vi "dfd_NStage MRate Set Filtering Mode.vi"(6 "filtering mode":T6=2 items=["No Rate Change", "Interpolation", "Decimation"], 8 "error in (no error)":errorcluster, 11 "multirate filter in":T1[](array[typedef]) {"mMRate_SumWl" min=1 max=32 step=1; "mMRate_InputIwl" min=1 max=32 step=1; "mMRate_GainWl" min=1 max=32 step=1; "mMRate_OutputWl" min=1 max=32 step=1; "mMRate_InputWl" min=1 max=32 step=1; "mMRate_CoefWl" min=1 max=32 step=1; "mMRate_Mode" items=["Default"=-1, "No Rate Change"=0, "Interpolation"=1, "Decimation"=2, "Interpolated"=3, "Rational"=4]}) -> (0 "error out":errorcluster, 3 "multirate filter out":T1[](array[typedef]) {"mMRate_SumWl" min=1 max=32 step=1; "mMRate_InputIwl" min=1 max=32 step=1; "mMRate_GainWl" min=1 max=32 step=1; "mMRate_OutputWl" min=1 max=32 step=1; "mMRate_InputWl" min=1 max=32 step=1; "mMRate_CoefWl" min=1 max=32 step=1; "mMRate_Mode" items=["Default"=-1, "No Rate Change"=0, "Interpolation"=1, "Decimation"=2, "Interpolated"=3, "Rational"=4]})   [LabVIEW 2017, in "NI_DigFilterLicensed.lvlib"]
uses:
  <vilib>/addons/Digital Filter Design/NI_DigFilterLicensed.lvlib
  <vilib>/addons/Digital Filter Design/_Objects.llb/DFD Multirate Filtering Mode.ctl
  <vilib>/addons/Digital Filter Design/_Objects.llb/DFD Multirate Filter Obj.ctl
  <vilib>/addons/Digital Filter Design/_Objects.llb/DFD Multirate Mode.ctl
  <vilib>/addons/Digital Filter Design/_Objects.llb/DFD Coef Norm Type.ctl
  <vilib>/addons/Digital Filter Design/_Objects.llb/DFD Round-off Mode.ctl
  <vilib>/addons/Digital Filter Design/_Objects.llb/DFD FXP MRate Multiply Mode.ctl
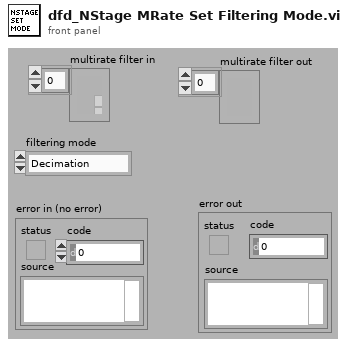
[diagram p1: front panel]
types:
  T1 = typedef "NI_DigFilterLicensed.lvlib/DFD Multirate Filter Obj.ctl" = cluster{"mMRate_Structure":enum16{"CIC", "FIR", "IIR", "Lattice"}, "mMRate_Mode":T2, "mMRate_Factor":i32, "mMRate_FIRParams":cluster{"mMRate_FIR_H":dbl[], "mMRate_FIR_IsNyquist?":bool, "mMRate_FIR_IsSymmetric?":bool}, "mMRate_CICParams":cluster{"mMRate_CIC_#Stage":i32, "mMRate_CIC_Lag":i32, "mMRate_CIC_Type":enum16{"Lowpass", "Highpass"}}, "mMRate_Order":i32, "mMRate_Version":string, "mMRate_Comments":string, "mMRate_RationalFactor":cluster{"mMRate_L":i32, "mMRate_M":i32}, "mMRate_Fs":dbl, "mMRate_Quantized?":bool, "mMRate_QFilterGain":dbl, "mMRate_CoefWl":i16, "mMRate_Scaling":cluster{"mMRate_ScaleByPowerOf2?":bool, "mMRate_ScaleType":T3}, "mMRate_InputWl":i16, "mMRate_OutputWl":i16, "mMRate_OutputMode":T4, "mMRate_MultMode":T5, "mMRate_BitPruning":bool, "mMRate_GainWl":i16, "mMRate_OutputFwl":i16, "mMRate_SumIwl":i16, "mMRate_InputIwl ":i16, "mMRate_SumWl":i16, "mMRate_CoefIwl":i16}
  T2 = typedef "NI_DigFilterLicensed.lvlib/DFD Multirate Mode.ctl" = i16
  T3 = typedef "NI_DigFilterLicensed.lvlib/DFD Coef Norm Type.ctl" = enum16{"No Norm", "Time Domain 1-Norm", "Time Domain 2-Norm", "Time Domain Inf-Norm"}
  T4 = typedef "NI_DigFilterLicensed.lvlib/DFD Round-off Mode.ctl" = enum16{"Nearest", "Truncation"}
  T5 = typedef "NI_DigFilterLicensed.lvlib/DFD FXP MRate Multiply Mode.ctl" = enum16{"Truncated", "Full"}
  T6 = typedef "NI_DigFilterLicensed.lvlib/DFD Multirate Filtering Mode.ctl" = u16
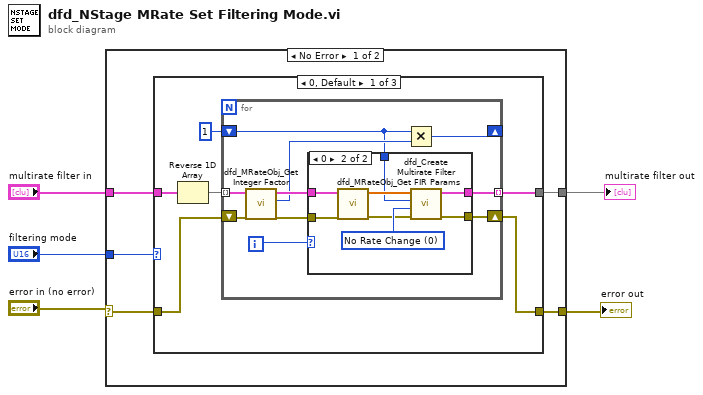
[diagram p0: block diagram]
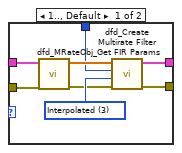
[diagram p2: hidden frame]
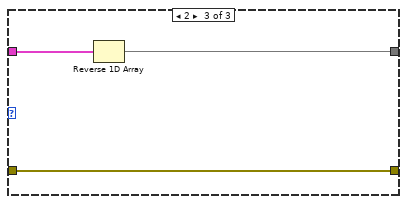
[diagram p4: hidden frame]
diagram:
  n1 = case shown="No Error" "error in (no error)" {
    selector: "error in (no error)" -> [w7 w45]
    tunnel: "filtering mode" -> [w10 _]
    tunnel: [w9 _] -> w4
    tunnel: "multirate filter in" -> [w8 _]
    tunnel: [w6 w45] -> w1
    frame No Error {
      n2 = case shown="0, Default" w10 {
        tunnel: w8 -> [w16 w41 w44]
        tunnel: [w12 w41 w43] -> w9
        tunnel: w7 -> [w14 w40 w42]
        tunnel: [w11 w40 w42] -> w6
        frame 0, Default {
          n3 = Reverse 1D Array(array=w16) -> (reversed array=w15:T1[])
          n4 = for {
            tunnel: w15 -> [w21] mode=indexing
            shift-right: [w18] -> _
            shift-left: 1 -> [w17]
            shift-right: [w23] -> w11
            shift-left: w14 -> [w24]
            tunnel: [w22] -> w12 mode=indexing
            i -> [w25]
            n5 = call <vilib>:"dfd_MRateObj_Get Integer Factor.vi"("multirate filter in"=w21) -> ("factor"=w19:i32, "dup multirate filter"=w20:T1)  [unwired: 9 out]
            n6 = case shown="0" w25 {
              tunnel: w20 -> [w32 w39]
              tunnel: w17 -> [w27 w34]
              tunnel: w24 -> [w26 w33]
              tunnel: [w30 w37] -> w23
              tunnel: [w29 w36] -> w22
              frame 1.., Default {
                w28 = T2 3 items=["Default"=-1, "No Rate Change"=0, "Interpolation"=1, "Decimation"=2, "Interpolated"=3] ("mode")
                n7 = call <vilib>:"dfd_MRateObj_Get FIR Params.vi"("multirate filter in"=w32) -> ("h(n)"=w31:dbl[])  [unwired: 1 in, 9 out]
                n8 = call <vilib>:"dfd_Create Multirate Filter.vi"("error in (no error)"=w26, "mode"=w28, "factor"=w27, "h (n)"=w31) -> ("error out"=w30:errorcluster, "multirate filter out"=w29:T1)  [unwired: 1 in, 5 out]
              }
              frame 0 {
                w35 = T2 0 items=["Default"=-1, "No Rate Change"=0, "Interpolation"=1, "Decimation"=2, "Interpolated"=3] ("mode")
                n9 = call <vilib>:"dfd_MRateObj_Get FIR Params.vi"("multirate filter in"=w39) -> ("h(n)"=w38:dbl[])  [unwired: 1 in, 9 out]
                n10 = call <vilib>:"dfd_Create Multirate Filter.vi"("error in (no error)"=w33, "mode"=w35, "factor"=w34, "h (n)"=w38) -> ("error out"=w37:errorcluster, "multirate filter out"=w36:T1)  [unwired: 1 in, 5 out]
              }
            }
            n11 = Multiply(x=w17, y=w19) -> (x*y=w18:i32)
          }
        }
        frame 1 {
        }
        frame 2 {
          n12 = Reverse 1D Array(array=w44) -> (reversed array=w43:T1[])
        }
      }
    }
    frame Error {
    }
  }
  "multirate filter out" <- w4
  "error out" <- w1
